vi "SetMatrixSub.vi"(1 "Array":bool[][](array[boolean])) -> ()   [LabVIEW 2017]
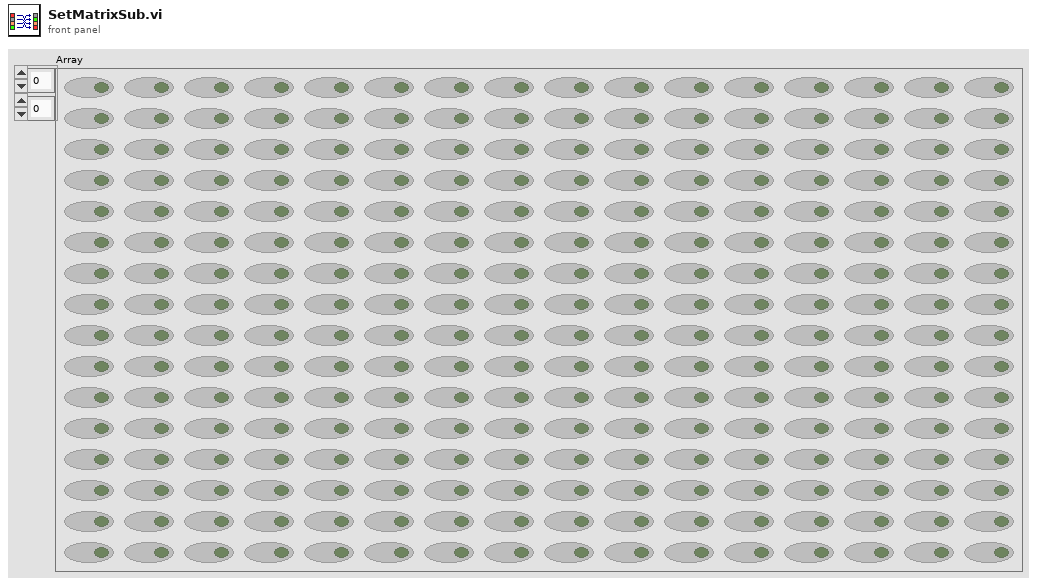
[diagram p1: front panel]
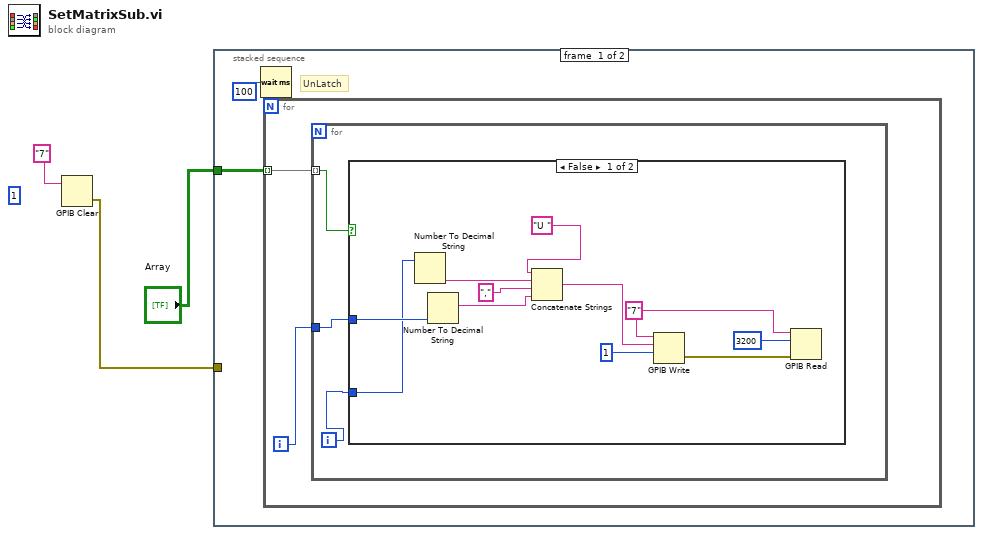
[diagram p0: block diagram]
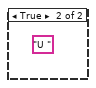
[diagram p2: hidden frame]
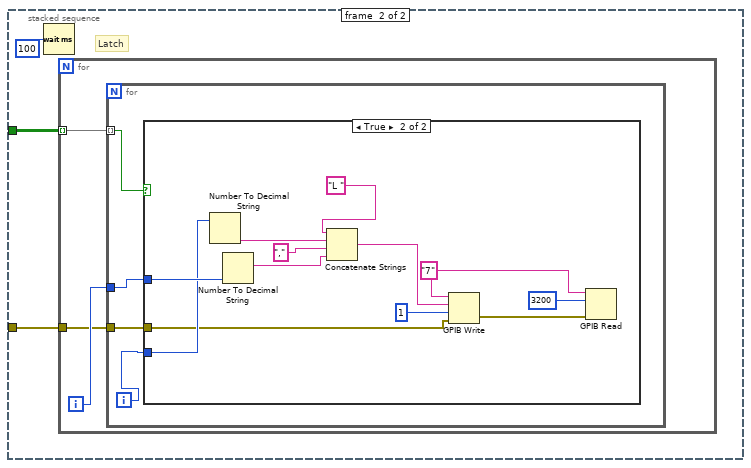
[diagram p3: hidden frame]
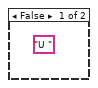
[diagram p4: hidden frame]
diagram:
  (unwired) 1
  n1 = GPIB Clear(3:"7") -> (0:w1:errorcluster)  [unwired: 1 in, 1 out]
  n2 = stacked-sequence {
    tunnel: "Array" -> [w5 w24]
    tunnel: w1 -> [_ w22]
    frame #0 {
      # "UnLatch"
      n3 = Wait (ms)(milliseconds to wait=100) -> ()  [unwired: 1 out]
      n4 = for {
        tunnel: w5 -> [w6] mode=indexing
        i -> [w7]
        n5 = for {
          tunnel: w7 -> [w9]
          tunnel: w6 -> [w10] mode=indexing
          i -> [w8]
          n6 = case shown="False" w10 {
            tunnel: w9 -> [w13 _]
            tunnel: w8 -> [w12 _]
            frame False {
              w16 = "7"
              n7 = Number To Decimal String(number=w12) -> (decimal integer string=w21:string)  [unwired: 1 in]
              n8 = Number To Decimal String(number=w13) -> (decimal integer string=w20:string)  [unwired: 1 in]
              n9 = Concatenate Strings("U ", w21, ",", w20) -> (w14:string)
              n10 = GPIB Write(0:w16, 1:w14, 2:1) -> (6:w18:errorcluster)  [unwired: 2 in, 1 out]
              n11 = GPIB Read(0:w16, 1:3200, 3:w18) -> ()  [unwired: 2 in, 3 out]
            }
            frame True {
              (unwired) "U "
            }
          }
        }
      }
    }
    frame #1 {
      # "Latch"
      n12 = Wait (ms)(milliseconds to wait=100) -> ()  [unwired: 1 out]
      n13 = for {
        tunnel: w24 -> [w26] mode=indexing
        tunnel: w22 -> [w25]
        i -> [w27]
        n14 = for {
          tunnel: w27 -> [w30]
          tunnel: w26 -> [w31] mode=indexing
          tunnel: w25 -> [w28]
          i -> [w29]
          n15 = case shown="True" w31 {
            tunnel: w30 -> [_ w35]
            tunnel: w29 -> [_ w34]
            tunnel: w28 -> [_ w32]
            frame False {
              (unwired) "U "
            }
            frame True {
              w38 = "7"
              n16 = Number To Decimal String(number=w34) -> (decimal integer string=w43:string)  [unwired: 1 in]
              n17 = Number To Decimal String(number=w35) -> (decimal integer string=w42:string)  [unwired: 1 in]
              n18 = Concatenate Strings("L ", w43, ",", w42) -> (w36:string)
              n19 = GPIB Write(0:w38, 1:w36, 2:1, 3:w32) -> (6:w40:errorcluster)  [unwired: 1 in, 1 out]
              n20 = GPIB Read(0:w38, 1:3200, 3:w40) -> ()  [unwired: 2 in, 3 out]
            }
          }
        }
      }
    }
  }
